vi "ROI entry-handle rectangle editing.vi"(8 "error in (no error)":errorcluster, 9 "Programatic event?":bool, 10 "Coordinates":i32[](array[numeric])) -> (0 "error IO":errorcluster, 1 "Cancelled":bool, 2 "ROIs Info []":T1[](array[typedef]) {"Zoom" min=1.0 max=10.0 step=0.10000000149011612})   [LabVIEW 2013]
uses:
  Typedefs/ROI spec.ctl
  Typedefs/ROI ID Enum.ctl
  ROI Entry screen/Globals/gl_ROI Entry UI globals.vi
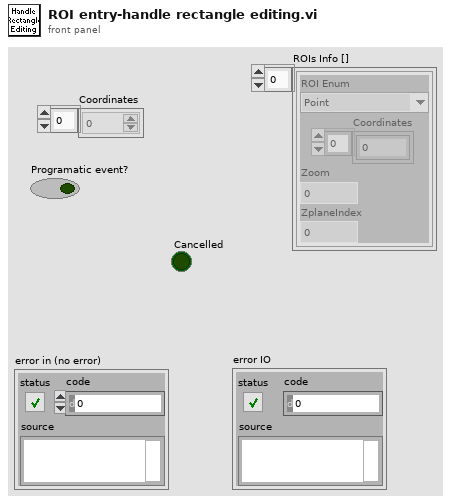
[diagram p1: front panel]
types:
  T1 = typedef "ROI spec.ctl" = cluster{"Coordinates":i32[], "Zoom":dbl, "ROI Enum":T2, "ZplaneIndex":i32}
  T2 = typedef "ROI ID Enum.ctl" = enum16{"Point", "MiniScan", "Comp. MiniScan", "Rectangle", "Comp. volume", "Arb. plane point"}
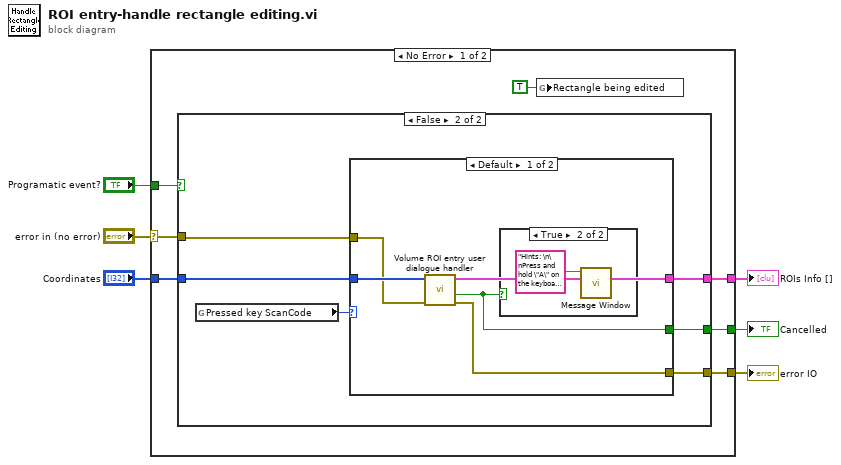
[diagram p0: block diagram]
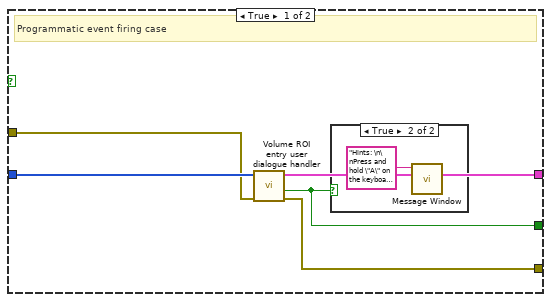
[diagram p2: hidden frame]
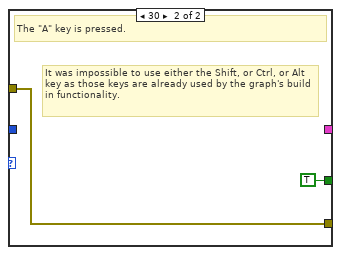
[diagram p5: hidden frame]
diagram:
  n1 = case shown="No Error" "error in (no error)" {
    selector: "error in (no error)" -> [w8 w34]
    tunnel: [w13 _] -> w6
    tunnel: "Coordinates" -> [w11 _]
    tunnel: [w10 _] -> w4
    tunnel: "Programatic event?" -> [w9 _]
    tunnel: [w7 w34] -> w2
    frame No Error {
      n2 = case shown="False" w9 {
        tunnel: [w15 w25] -> w13
        tunnel: w11 -> [w18 w24]
        tunnel: [w17 w23] -> w10
        tunnel: w8 -> [w16 w21]
        tunnel: [w14 w20] -> w7
        frame True {
          # "Programmatic event firing case"
          n3 = call "Volume ROI entry user dialogue handler.vi"("error in (no error)"=w16, "New coordinates"=w18) -> ("error IO"=w14:errorcluster, "Cancelled"=w15:bool, "ROIs Info []"=w17:T1[])  [unwired: 7 in]
          n4 = case shown="True" w15 {
            frame False {
            }
            frame True {
              n5 = call "Message Window.vi"("Message string"="Hints: \n\nPress and hold \"A\" on the keyboard while editing the rectangle to prevent the previous window constantly popping up.\n\nHold down the \"Shift\" key to restrict the rotation to 45 degree increments. \n\nTo use both keys simultaneously press and hold \"Shift\" before pressing the \"A\" key.") -> ()  [unwired: 10 in, 1 out]
            }
          }
        }
        frame False {
          n6 = global read "gl_ROI Entry UI globals.vi" "Pressed key ScanCode"() -> (w22:i16)
          n7 = case shown="Default" w22 {
            tunnel: [w30 _] -> w23
            tunnel: w24 -> [w29 _]
            tunnel: [w27 TRUE ("Cancelled")] -> w25
            tunnel: w21 -> [w28 w32]
            tunnel: [w26 w32] -> w20
            frame Default {
              n8 = call "Volume ROI entry user dialogue handler.vi"("error in (no error)"=w28, "New coordinates"=w29) -> ("error IO"=w26:errorcluster, "Cancelled"=w27:bool, "ROIs Info []"=w30:T1[])  [unwired: 7 in]
              n9 = case shown="True" w27 {
                frame False {
                }
                frame True {
                  n10 = call "Message Window.vi"("Message string"="Hints: \n\nPress and hold \"A\" on the keyboard while editing the rectangle to prevent the previous window constantly popping up.\n\nHold down the \"Shift\" key to restrict the rotation to 45 degree increments. \n\nTo use both keys simultaneously press and hold \"Shift\" before pressing the \"A\" key.") -> ()  [unwired: 10 in, 1 out]
                }
              }
            }
            frame 30 {
              # "It was impossible to use either the Shift, or Ctrl, or Alt key as those keys are already used by the graph's build in functionality."
              # "The \"A\" key is pressed."
            }
          }
        }
      }
      n11 = global write "gl_ROI Entry UI globals.vi" "Rectangle being edited"(TRUE ("Rectangle being edited")) -> ()
    }
    frame Error {
    }
  }
  "Cancelled" <- w6
  "ROIs Info []" <- w4
  "error IO" <- w2
